vi "scancode to number.vi"(10 "keypad code":i32) -> (2 "keypad value":i32)   [LabVIEW 2013]
panel:
  # "scancode to number"
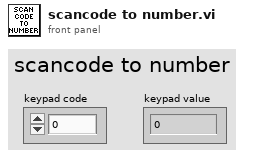
[diagram p1: front panel]
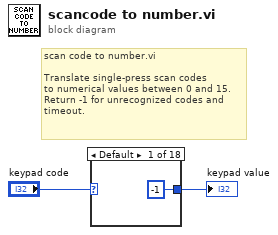
[diagram p0: block diagram]
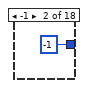
[diagram p2: hidden frame]
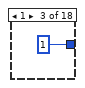
[diagram p3: hidden frame]
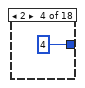
[diagram p4: hidden frame]
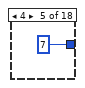
[diagram p5: hidden frame]
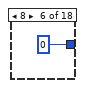
[diagram p6: hidden frame]
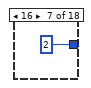
[diagram p7: hidden frame]
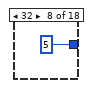
[diagram p8: hidden frame]
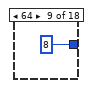
[diagram p9: hidden frame]
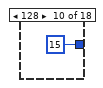
[diagram p10: hidden frame]
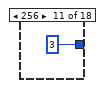
[diagram p11: hidden frame]
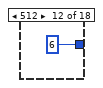
[diagram p12: hidden frame]
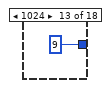
[diagram p13: hidden frame]
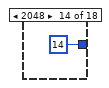
[diagram p14: hidden frame]
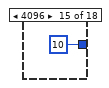
[diagram p15: hidden frame]
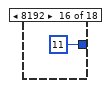
[diagram p16: hidden frame]
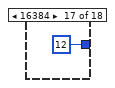
[diagram p17: hidden frame]
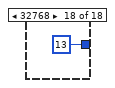
[diagram p18: hidden frame]
diagram:
  # "scan code to number.vi\n\nTranslate single-press scan codes\nto numerical values between 0 and 15.\nReturn -1 for unrecognized codes and\ntimeout."
  n1 = case shown="Default" "keypad code" {
    tunnel: [-1 ("keypad code") -1 ("keypad code") 1 4 7 0 2 5 8 15 3 6 9 14 10 11 12 13] -> w1
    frame Default {
    }
    frame -1 {
    }
    frame 1 {
    }
    frame 2 {
    }
    frame 4 {
    }
    frame 8 {
    }
    frame 16 {
    }
    frame 32 {
    }
    frame 64 {
    }
    frame 128 {
    }
    frame 256 {
    }
    frame 512 {
    }
    frame 1024 {
    }
    frame 2048 {
    }
    frame 4096 {
    }
    frame 8192 {
    }
    frame 16384 {
    }
    frame 32768 {
    }
  }
  "keypad value" <- w1
